vi "setVel.vi"(1 "vel (mm/s)":dbl=10.0, 2 "input cluster":T1) -> (0 "Controller error":bool)   [LabVIEW 2015]
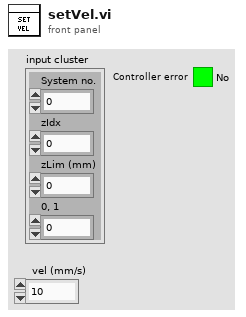
[diagram p1: front panel]
types:
  T1 = cluster{"System no.":i32, "zIdx":i32, "zLim (mm)":dbl, "0, 1":i16}
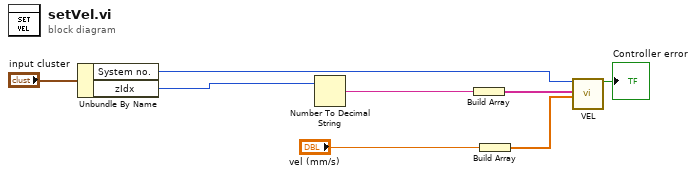
[diagram p0: block diagram]
diagram:
  n1 = Unbundle By Name("input cluster") -> ("System no."=w3:i32, "zIdx"=w7:i32)
  n2 = Number To Decimal String(number=w7) -> (decimal integer string=w6:string)  [unwired: 1 in]
  n3 = Build Array(w6) -> (w8:string[])
  n4 = Build Array("vel (mm/s)") -> (w5:dbl[])
  n5 = call "VEL.vi"("System no."=w3, "Axes to set"=w8, "Velocity values"=w5) -> ("Controller error"=→"Controller error":bool)  [unwired: 15 in, 1 out]
